vi "Disabled channel logic 4ch.vi"(7 "reset":bool, 9 "input valid":bool, 10 "data":u32[](array[numeric])=[0, 0, 0, 0], 11 "enabled channels":u32) -> (1 "data ready":bool, 2 "data out":u32[](array[numeric]))   [LabVIEW 2025, in "niUSRP Stream Control (DMA) v1 FPGA.lvclass"]
uses:
  niUSRP Stream Control (DMA) v1 FPGA.lvclass
  niUSRP Stream Control (DMA) v1 FPGA.lvclass/niUSRP Stream Control (DMA) v1 FPGA.ctl
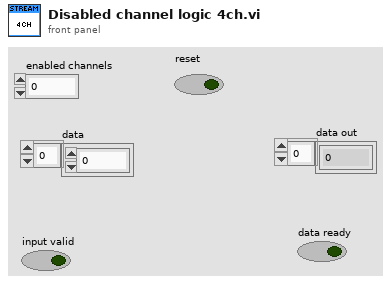
[diagram p1: front panel]
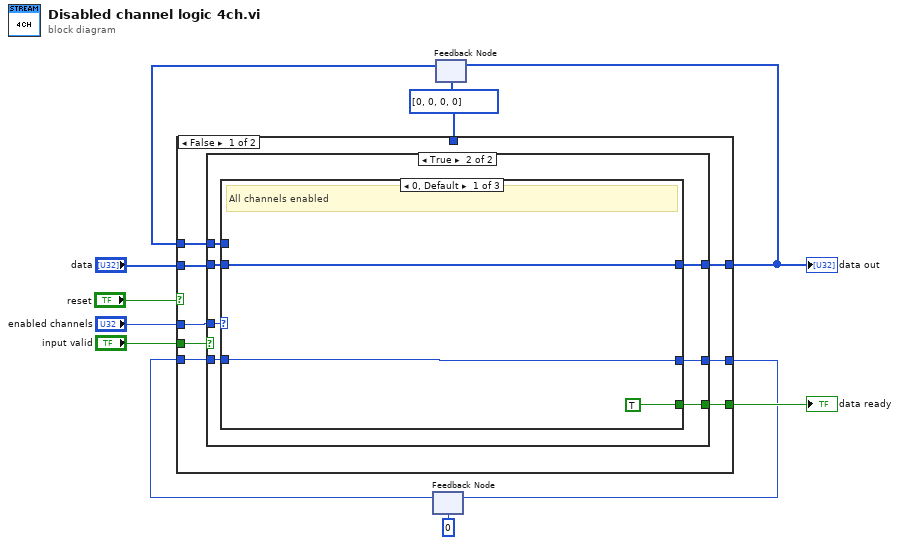
[diagram p0: block diagram]
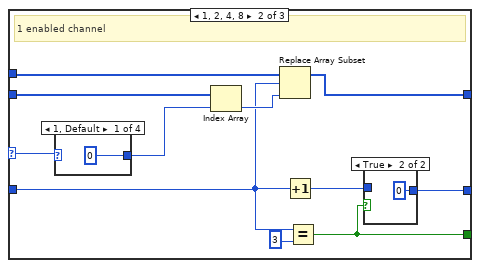
[diagram p3: hidden frame]
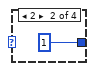
[diagram p5: hidden frame]
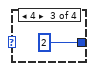
[diagram p6: hidden frame]
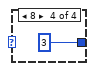
[diagram p7: hidden frame]
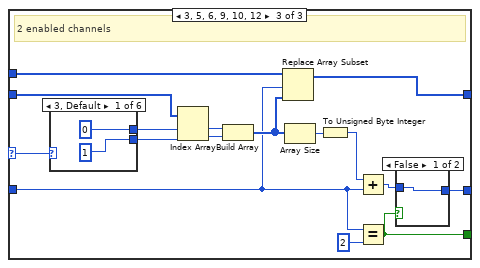
[diagram p8: hidden frame]
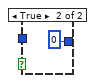
[diagram p9: hidden frame]
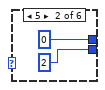
[diagram p10: hidden frame]
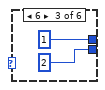
[diagram p11: hidden frame]
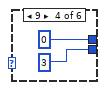
[diagram p12: hidden frame]
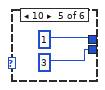
[diagram p13: hidden frame]
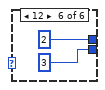
[diagram p14: hidden frame]
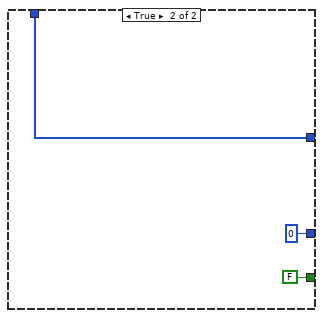
[diagram p15: hidden frame]
diagram:
  w1 = u32[] [0, 0, 0, 0]
  n1 = feedback #1(u8 0) -> (w3:u8)
  n2 = feedback #2(w1) -> (w11:u32[])
  n3 = case shown="False" "reset" {
    tunnel: w11 -> [w19 _]
    tunnel: "enabled channels" -> [w18 _]
    tunnel: "data" -> [w17 _]
    tunnel: [w16 w80] -> w8
    tunnel: [w15 FALSE] -> w7
    tunnel: "input valid" -> [w14 _]
    tunnel: [w13 u8 0] -> w4
    tunnel: w3 -> [w12 _]
    tunnel: w1 -> [_ w80]
    frame False {
      n4 = case shown="True" w14 {
        selector: w14 -> [w20 _]
        tunnel: [w22 w29] -> w16
        tunnel: w19 -> [w22 w28]
        tunnel: w17 -> [_ w27]
        tunnel: w18 -> [_ w26]
        tunnel: [w21 w25] -> w13
        tunnel: w12 -> [w21 w24]
        tunnel: [w20 w23] -> w15
        frame False {
        }
        frame True {
          n5 = case shown="0, Default" w26 {
            selector: w26 -> [_ w39 w64]
            tunnel: w27 -> [w32 w41 w54]
            tunnel: [w32 w42 w61] -> w29
            tunnel: [TRUE w35 w50] -> w23
            tunnel: w24 -> [w31 w36 w53]
            tunnel: [w31 w33 w51] -> w25
            tunnel: w28 -> [_ w40 w60]
            frame 0, Default {
              # "All channels enabled"
            }
            frame 1, 2, 4, 8 {
              # "1 enabled channel"
              n6 = case shown="1, Default" w39 {
                tunnel: [0 ("index") 1 ("index") 2 ("index") 3 ("index")] -> w38
                frame 1, Default {
                }
                frame 2 {
                }
                frame 4 {
                }
                frame 8 {
                }
              }
              n7 = Index Array(array=w41, index=w38) -> (element=w37:u32)
              n8 = Replace Array Subset(array=w40, new element=w37, index=w36) -> (w42:u32[])
              n9 = Increment(x=w36) -> (x+1=w34:u8)
              n10 = Equal?(x=w36, y=u8 3) -> (x = y?=w35:bool)
              n11 = case shown="True" w35 {
                tunnel: [w44 u8 0] -> w33
                tunnel: w34 -> [w44 _]
                frame False {
                }
                frame True {
                }
              }
            }
            frame 3, 5, 6, 9, 10, 12 {
              # "2 enabled channels"
              n12 = case shown="3, Default" w64 {
                tunnel: [0 ("index") 0 ("index") 1 ("index") 0 ("index") 1 ("index") 2 ("index")] -> w56
                tunnel: [1 ("index") 2 ("index") 2 ("index") 3 ("index") 3 ("index") 3 ("index")] -> w55
                frame 3, Default {
                }
                frame 5 {
                }
                frame 6 {
                }
                frame 9 {
                }
                frame 10 {
                }
                frame 12 {
                }
              }
              n13 = Index Array(array=w54, index #1=w56, index #2=w55) -> (element #1=w59:u32, element #2=w58:u32)
              n14 = Build Array(w59, w58) -> (w57:u32[])
              n15 = Replace Array Subset(array=w60, new element=w57, index=w53) -> (w61:u32[])
              n16 = Array Size(array=w57) -> (size(s)=w63:i32)
              n17 = To Unsigned Byte Integer(number=w63) -> (unsigned 8bit integer=w62:u8)
              n18 = Add(x=w62, y=w53) -> (x+y=w52:u8)
              n19 = Equal?(x=w53, y=u8 2) -> (x = y?=w50:bool)
              n20 = case shown="False" w50 {
                tunnel: [w66 u8 0] -> w51
                tunnel: w52 -> [w66 _]
                frame False {
                }
                frame True {
                }
              }
            }
          }
        }
      }
    }
    frame True {
    }
  }
  "data out" <- w8
  "data ready" <- w7
  n21 = feedback-in #1(w4) -> ()
  n22 = feedback-in #2(w8) -> ()
